vi "Gamma Ai.vi"(1 "Yi(t)":dbl, 2 "V":dbl, 3 "U":dbl, 4 "H":dbl) -> (0 "Gamma ai":dbl)   [LabVIEW 2012]
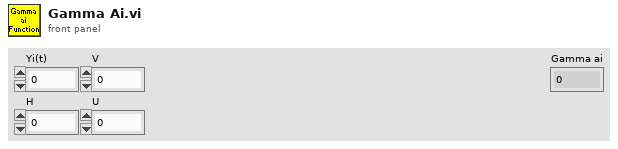
[diagram p1: front panel]
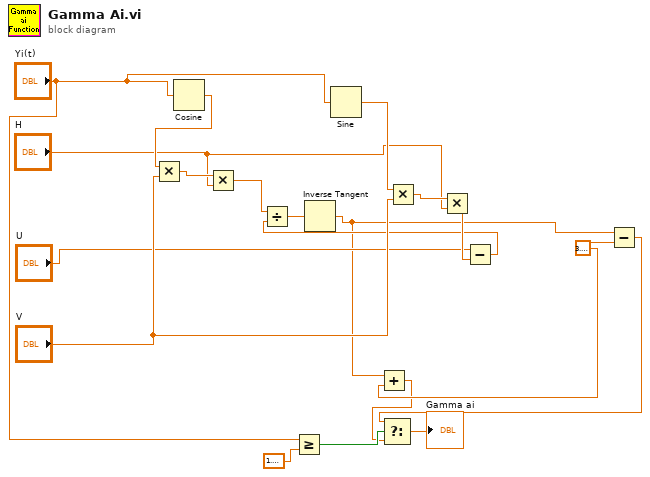
[diagram p0: block diagram]
diagram:
  w3 = 3.141592653589793
  n1 = Cosine(x="Yi(t)") -> (cos(x)=w19:dbl)
  n2 = Multiply(x=w19, y="V") -> (x*y=w18:dbl)
  n3 = Multiply(x=w18, y="H") -> (x*y=w11:dbl)
  n4 = Greater Or Equal?(x="Yi(t)", y=1.5707963267948966) -> (x >= y?=w6:bool)
  n5 = Sine(x="Yi(t)") -> (sin(x)=w16:dbl)
  n6 = Multiply(x=w16, y="V") -> (x*y=w17:dbl)
  n7 = Multiply(x=w17, y="H") -> (x*y=w13:dbl)
  n8 = Subtract(x="U", y=w13) -> (x-y=w10:dbl)
  n9 = Divide(x=w11, y=w10) -> (x/y=w9:dbl)
  n10 = Inverse Tangent(1:w9) -> (0:w4:dbl)
  n11 = Add(x=w4, y=w3) -> (x+y=w2:dbl)
  n12 = Subtract(x=w4, y=w3) -> (x-y=w5:dbl)
  n13 = Select(t=w5, s=w6, f=w2) -> (s? t:f=→"Gamma ai":dbl)
